vi "svmdense_get_libsvm_version.vi"(8 "error in (no error)":errorcluster) -> (0 "error out":errorcluster, 3 "version":i32)   [LabVIEW 2015]
uses:
  bin/x64/LabVIEW-libsvm-dense.dll
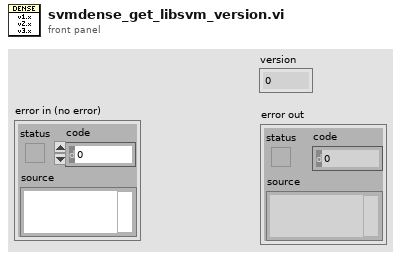
[diagram p1: front panel]
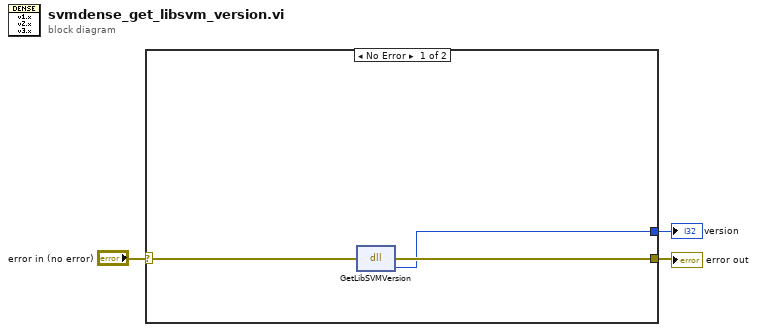
[diagram p0: block diagram]
diagram:
  n1 = case shown="No Error" "error in (no error)" {
    selector: "error in (no error)" -> [w6 w7]
    tunnel: [w5 w7] -> w3
    tunnel: [w4 _] -> w1
    frame No Error {
      n2 = dll-call lib="C:/dev/LabVIEW-libsvm/LabVIEW/bin/x64/LabVIEW-libsvm-dense.dll" fn="GetLibSVMVersion"(error in=w6) -> (error out=w5:errorcluster, "return type"=w4:i32)  [unwired: 2 in, 1 out]
    }
    frame Error {
    }
  }
  "error out" <- w3
  "version" <- w1
